vi "SVT Dynamic Range (Frequency) (1 Ch).vi"(0 "complex spectrum":T7={"complex spectrum response"={"f0"=0.0, "df"=1.0, "complex spectrum"=[]}, "spectrum info"={"channel name"="", "description"="", "x-axis units"=0, "spectral info"={"spectrum type"=enum."Power [Magnitude^2]", "linear/dB"=enum."linear", "window"=0, "window size"=0, "FFT size"=0}, "engineering units"=0, "custom label"="", "dB reference [EU]"=0.0, "peak units"=enum."rms", "weighting filter"=0, "spectral density?"=FALSE, "unit label"="", "spectrum skewed?"=FALSE, "complimentary spectrum units"=enum."none"}} {"spectrum info"."x-axis units" items=["Time (s)"=0, "Frequency-CB (Hz)"=1, "Frequency-CPB (Hz)"=1248, "Frequency-Arbitrary (Hz)"=2357, "Quefrency (s)"=2, "Revolutions (rev)"=3, "Order"=4, "Speed (RPM)"=11, "Speed (rad/s)"=21, "Index"=65535]; "spectrum info"."weighting filter" items=["Linear", "A-weighting", "B-weighting", "C-weighting", "ITU-R 468-4", "Dolby", "CCITT", "C-message", "Wb", "Wc", "Wd", "We", "Wf", "Wh", "Wj", "Wk", "Wm", "AES17 20 kHz lowpass", "AES17 40 kHz lowpass", "AES17 20 kHz highpass", "AES17 40 kHz highpass"]; "spectrum info"."dB reference [EU]" format="%.2f"; "spectrum info"."engineering units" items=["custom..."=0, "V"=1, "A"=21, "C"=30, "pC"=31, "s"=32, "-"=29, "Pa"=2, "N"=20, "g"=3, "m/s^2"=4, "m/s"=5, "m"=6, "mm/s"=12, "mm"=13, "micron/s"=14, "micron"=15, "in/s^2"=7, "in/s"=8, "in"=9, "mil/s"=10, "mil"=11, "rad/s^2"=16, "rad/s"=17, "rad"=18, "deg/s^2"=26, "deg/s"=27, "deg"=28, "RPM"=22, "cycle/s^2"=23, "Hz"=24, "cycle"=25, "strain"=19]; "spectrum info"."spectral info"."window" items=["None "=0, "Hanning"=1, "Hamming"=2, "Blackman-Harris"=3, "Exact Blackman"=4, "Blackman"=5, "Flat Top"=6, "4 Term B-Harris "=7, "7 Term B-Harris"=8, "Low Sidelobe"=9, "Force - Exponential"=10, "Gaussian"=62]; "complex spectrum response"."complex spectrum" format="%.2f"; "complex spectrum response"."df" format="%.2f"; "complex spectrum response"."f0" format="%.2f"}, 2 "frequency range":T10={"start frequency"=-1.0, "stop frequency"=-1.0} {"stop frequency" format="%.2f"; "start frequency" format="%.2f"}, 3 "advanced span [Hz]":dbl=-1.0 format="%.2f", 5 "error in (no error)":errorcluster, 6 "desired units":T9={"dynamic range units"=enum."dB", "detected fundamental amplitude units"=enum."EU peak"}, 7 "full scale amplitude [EU peak]":dbl=10.0 format="%.2f", 9 "expected fundamental\nfrequency [Hz]":dbl=-1.0 format="%.2f") -> (11 "detected fundamental\nfrequency [Hz]":dbl=nan format="%.2f", 12 "unit labels":T8, 13 "detected fundamental\namplitude":dbl=nan format="%.2f", 14 "dup complex spectrum":T7={"complex spectrum response"={"f0"=0.0, "df"=1.0, "complex spectrum"=[]}, "spectrum info"={"channel name"="", "description"="", "x-axis units"=0, "spectral info"={"spectrum type"=enum."Power [Magnitude^2]", "linear/dB"=enum."linear", "window"=0, "window size"=0, "FFT size"=0}, "engineering units"=0, "custom label"="", "dB reference [EU]"=0.0, "peak units"=enum."rms", "weighting filter"=0, "spectral density?"=FALSE, "unit label"="", "spectrum skewed?"=FALSE, "complimentary spectrum units"=enum."none"}} {"spectrum info"."x-axis units" items=["Time (s)"=0, "Frequency-CB (Hz)"=1, "Frequency-CPB (Hz)"=1248, "Frequency-Arbitrary (Hz)"=2357, "Quefrency (s)"=2, "Revolutions (rev)"=3, "Order"=4, "Speed (RPM)"=11, "Speed (rad/s)"=21, "Index"=65535]; "spectrum info"."weighting filter" items=["Linear", "A-weighting", "B-weighting", "C-weighting", "ITU-R 468-4", "Dolby", "CCITT", "C-message", "Wb", "Wc", "Wd", "We", "Wf", "Wh", "Wj", "Wk", "Wm", "AES17 20 kHz lowpass", "AES17 40 kHz lowpass", "AES17 20 kHz highpass", "AES17 40 kHz highpass"]; "spectrum info"."dB reference [EU]" format="%.2f"; "spectrum info"."engineering units" items=["custom..."=0, "V"=1, "A"=21, "C"=30, "pC"=31, "s"=32, "-"=29, "Pa"=2, "N"=20, "g"=3, "m/s^2"=4, "m/s"=5, "m"=6, "mm/s"=12, "mm"=13, "micron/s"=14, "micron"=15, "in/s^2"=7, "in/s"=8, "in"=9, "mil/s"=10, "mil"=11, "rad/s^2"=16, "rad/s"=17, "rad"=18, "deg/s^2"=26, "deg/s"=27, "deg"=28, "RPM"=22, "cycle/s^2"=23, "Hz"=24, "cycle"=25, "strain"=19]; "spectrum info"."spectral info"."window" items=["None "=0, "Hanning"=1, "Hamming"=2, "Blackman-Harris"=3, "Exact Blackman"=4, "Blackman"=5, "Flat Top"=6, "4 Term B-Harris "=7, "7 Term B-Harris"=8, "Low Sidelobe"=9, "Force - Exponential"=10, "Gaussian"=62]; "complex spectrum response"."complex spectrum" format="%.2f"; "complex spectrum response"."df" format="%.2f"; "complex spectrum response"."f0" format="%.2f"}, 16 "dynamic range":dbl=nan format="%.2f", 19 "error out":errorcluster)   [LabVIEW 2017, in "SoundVib_SingleTone.lvlib"]
doc: "Computes the dynamic range of a channel based on<B> scaled signal</B> and <B>full scale amplitude</B> and returns the detected fundamental frequency, detected fundamental amplitude, and dynamic range. This VI does not maintain state internally; you can use this VI in a loop to process multiple blocks. Wire data to the <B>scaled signal [EU]</B> input to determine the polymorphic instance to use or manually select the instance."
uses:
  <vilib>/addons/Sound and Vibration/svt_Single Tone Measurements/SoundVib_SingleTone.lvlib
  <vilib>/addons/_NISVFA/_Shared subVIs/Controls/svc_Spectrum Info.ctl
  <vilib>/addons/_NISVFA/_Shared subVIs/Controls/svc_X-Axis Units.ctl
  <vilib>/addons/_NISVFA/_Shared subVIs/Controls/svc_Spectrum Type.ctl
  <vilib>/addons/_NISVFA/_Shared subVIs/Controls/svc_Engineering Units Text Ring.ctl
  <vilib>/addons/_NISVFA/_Shared subVIs/Controls/svc_Weighting Filter Text Ring.ctl
  <vilib>/addons/_NISVFA/_Shared subVIs/Controls/svc_Complimentary Spectrum Units.ctl
  <vilib>/addons/Sound and Vibration/svt_Distortion/SoundVib_Distortion.lvlib
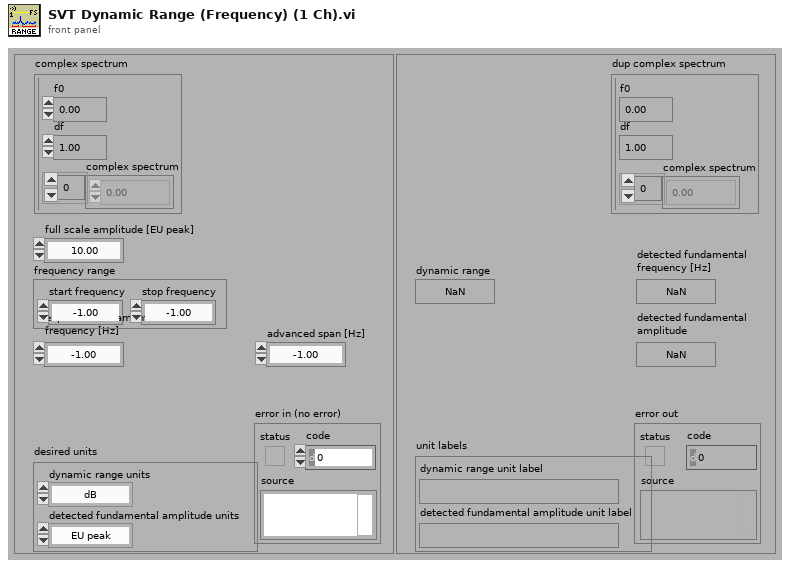
[diagram p1: front panel]
types:
  T1 = typedef "svc_Spectrum Info.ctl" = cluster{"channel name":string, "description":string, "x-axis units":T2, "spectral info":cluster{"spectrum type":T3, "linear/dB":enum16{"linear", "dB"}, "window":u16, "window size":i32, "FFT size":i32}, "engineering units":T4, "custom label":string, "dB reference [EU]":dbl, "peak units":enum16{"rms", "peak", "peak-peak"}, "weighting filter":T5, "spectral density?":bool, "unit label":string, "spectrum skewed?":bool, "complimentary spectrum units":T6}
  T2 = typedef "svc_X-Axis Units.ctl" = u16
  T3 = typedef "svc_Spectrum Type.ctl" = enum16{"FFT Spectrum [complex]", "Amplitude [Magnitude]", "Power [Magnitude^2]", "Cross Spectrum [complex]", "Frequency Response [Complex]"}
  T4 = typedef "svc_Engineering Units Text Ring.ctl" = u16
  T5 = typedef "svc_Weighting Filter Text Ring.ctl" = u16
  T6 = typedef "svc_Complimentary Spectrum Units.ctl" = enum16{"none", "radians", "degrees", "cycles", "imaginary"}
  T7 = cluster{"complex spectrum response":cluster{"f0":dbl, "df":dbl, "complex spectrum":cdb[]}, "spectrum info":T1}
  T8 = cluster{"dynamic range unit label":string, "detected fundamental amplitude unit label":string}
  T9 = cluster{"dynamic range units":enum16{"dB", "ENOB"}, "detected fundamental amplitude units":enum16{"EU rms", "EU peak", "EU peak-peak"}}
  T10 = cluster{"start frequency":dbl, "stop frequency":dbl}
  T11 = cluster{"SINAD unit label":string, "fundamental amplitude unit label":string}
  T12 = cluster{"SINAD units":enum16{"dB", "linear ratio", "%"}, "detected amplitude units":enum16{"EU rms", "EU peak", "EU peak-peak"}}
  T13 = cluster{"SINAD unit label":string, "detected fundamental amplitude unit label":string}
  T14 = cluster{"unit label":string, "unit label":string}
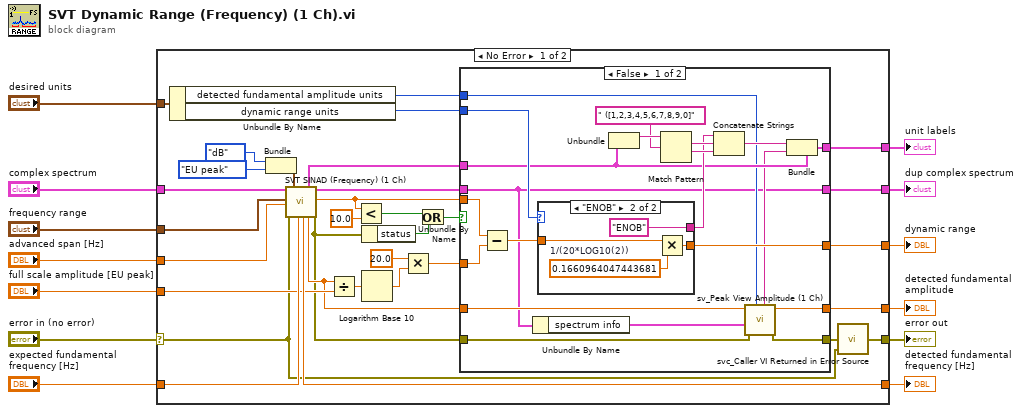
[diagram p0: block diagram]
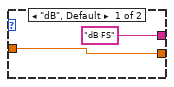
[diagram p2: hidden frame]
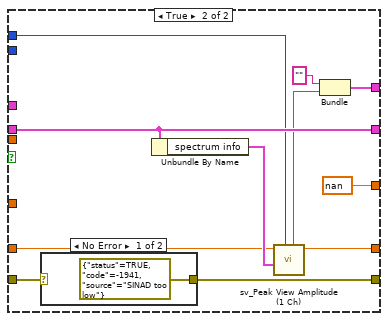
[diagram p3: hidden frame]
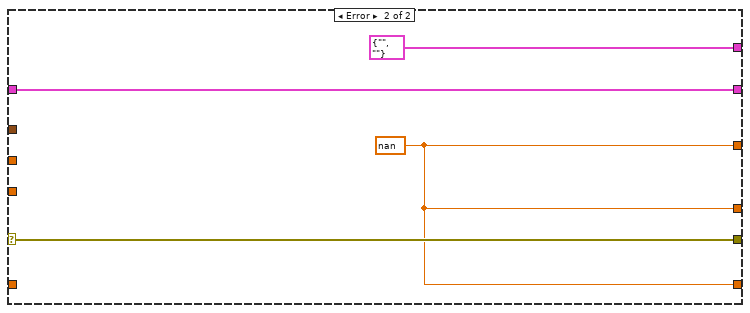
[diagram p5: hidden frame]
diagram:
  n1 = case shown="No Error" "error in (no error)" {
    selector: "error in (no error)" -> [w14 w89]
    tunnel: "full scale amplitude [EU peak]" -> [w41 _]
    tunnel: [w33 w88] -> w12
    tunnel: [w21 w89] -> w11
    tunnel: "complex spectrum" -> [w45 w86]
    tunnel: "expected fundamental\nfrequency [Hz]" -> [w44 _]
    tunnel: "desired units" -> [w38 _]
    tunnel: [w20 w86] -> w6
    tunnel: "frequency range" -> [w43 _]
    tunnel: [w30 w88] -> w4
    tunnel: [w42 w88] -> w3
    tunnel: [w32 T11 {"SINAD unit label"="", "fundamental amplitude unit label"=""} ("unit labels")] -> w2
    tunnel: "advanced span [Hz]" -> [w15 _]
    frame No Error {
      n2 = Unbundle By Name(w38) -> ("detected fundamental amplitude units"=w25:enum16{"EU rms", "EU peak", "EU peak-peak"}, "dynamic range units"=w34:enum16{"dB", "ENOB"})
      n3 = Bundle("SINAD units"=enum16{"dB", "linear ratio", "%"}."dB", "detected amplitude units"=enum16{"EU rms", "EU peak", "EU peak-peak"}."EU peak") -> (w37:T12)  [unwired: 1 in]
      n4 = call <vilib>:"SVT SINAD (Frequency) (1 Ch).vi"("complex spectrum"=w45, "frequency range"=w43, "advanced span [Hz]"=w15, "error in (no error)"=w14, "desired units"=w37, "expected fundamental frequency [Hz]"=w44) -> ("detected fundamental\nfrequency [Hz]"=w42:dbl, "unit labels"=w31:T13, "detected fundamental\namplitude"=w29:dbl, "complex spectrum"=w26:T7, "SINAD"=w24:dbl, "error out"=w19:errorcluster)  [unwired: 8 in]
      n5 = Divide(x=w29, y=w41) -> (x/y=w40:dbl)
      n6 = Less?(x=w24, y=10.0) -> (x < y?=w18:bool)
      n7 = Unbundle By Name(w19) -> ("status"=w17:bool)
      n8 = Logarithm Base 10(1:w40) -> (0:w39:dbl)
      n9 = Multiply(x=20.0 ("y"), y=w39) -> (x*y=w27:dbl)
      n10 = Or(x=w18, y=w17) -> (x .or. y?=w16:bool)
      n11 = case shown="False" w16 {
        tunnel: w34 -> [w66 _]
        tunnel: [w64 nan] -> w33
        tunnel: [w63 w74] -> w32
        tunnel: w31 -> [w56 _]
        tunnel: [w55 w77] -> w30
        tunnel: w29 -> [w54 w79]
        tunnel: w19 -> [w53 w83]
        tunnel: w27 -> [w52 _]
        tunnel: w26 -> [w46 w80]
        tunnel: w25 -> [w50 w78]
        tunnel: w24 -> [w48 _]
        tunnel: [w47 w82] -> w22
        tunnel: [w46 w80] -> w20
        frame False {
          n12 = Subtract(x=w48, y=w52) -> (x-y=w65:dbl)
          n13 = Unbundle By Name(w46) -> ("spectrum info"=w51:T1)
          n14 = case shown="\"ENOB\"" w66 {
            tunnel: [w68 w72] -> w64
            tunnel: w65 -> [w68 w71]
            tunnel: ["dB FS" ("fundamental amplitude unit label") "ENOB" ("fundamental amplitude unit label")] -> w58
            frame "dB", Default {
            }
            frame "ENOB" {
              w70 = 0.1660964047443681  # 1/(20*LOG10(2))
              n15 = Multiply(x=w71, y=w70) -> (x*y=w72:dbl)
            }
          }
          n16 = Unbundle(w56) -> ("SINAD unit label"=w62:string)  [unwired: 1 out]
          n17 = Match Pattern(string=w62, regular expression=" ([1,2,3,4,5,6,7,8,9,0]") -> (match substring=w60:string, after substring=w59:string)  [unwired: 1 in, 2 out]
          n18 = Concatenate Strings(w58, w60, w59) -> (w57:string)
          n19 = call <vilib>:"sv_Peak View Amplitude (1 Ch).vi"("peak units"=w50, "error in (no error)"=w53, "spectrum info"=w51, "peak amplitude [EU pk]"=w54) -> ("error out"=w47:errorcluster, "converted peak amplitude"=w55:dbl, "unit label"=w49:string)  [unwired: 5 in]
          n20 = Bundle(cluster=w56, "SINAD unit label"=w57, "detected fundamental amplitude unit label"=w49) -> (w63:T13)
        }
        frame True {
          n21 = case shown="No Error" w83 {
            selector: w83 -> [_ w85]
            tunnel: [errorcluster {"status"=TRUE, "code"=-1941, "source"="SINAD too low"} ("error IO") w85] -> w82
            frame No Error {
            }
            frame Error {
            }
          }
          n22 = Unbundle By Name(w80) -> ("spectrum info"=w81:T1)
          n23 = call <vilib>:"sv_Peak View Amplitude (1 Ch).vi"("peak units"=w78, "spectrum info"=w81, "peak amplitude [EU pk]"=w79) -> ("converted peak amplitude"=w77:dbl, "unit label"=w75:string)  [unwired: 6 in, 1 out]
          n24 = Bundle("unit label"="", "unit label"=w75) -> (w74:T14)  [unwired: 1 in]
        }
      }
      n25 = call <vilib>:"svc_Caller VI Returned in Error Source.vi"("warning input to caller"=w14, "error in (no error)"=w22) -> ("error out"=w21:errorcluster)  [unwired: 3 in]
    }
    frame Error {
      w88 = nan
    }
  }
  "dynamic range" <- w12
  "error out" <- w11
  "unit labels" <- w2
  "dup complex spectrum" <- w6
  "detected fundamental\nfrequency [Hz]" <- w3
  "detected fundamental\namplitude" <- w4
